vi "SGP Calculator.vi"(8 "End Flow":dbl, 9 "Flow Array":dbl[](array[numeric]), 10 "Start Index":i32, 11 "Resistance":dbl) -> (0 "End Flow Out":dbl, 2 "SGP":dbl, 3 "Start Flow":dbl)   [LabVIEW 2018, in "AnalysisSupport.lvlib"]
uses:
  AnalysisSupport.lvlib
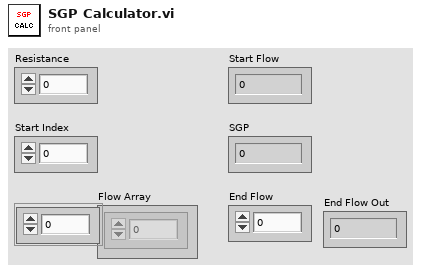
[diagram p1: front panel]
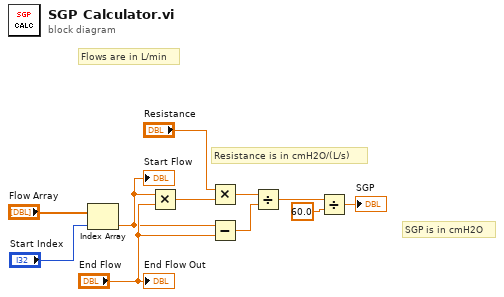
[diagram p0: block diagram]
diagram:
  # "Flows are in L/min"
  # "SGP is in cmH2O"
  # "Resistance is in cmH2O/(L/s)"
  n1 = Index Array(array="Flow Array", index="Start Index") -> (element=w8:dbl)
  "Start Flow" <- w8
  n2 = Multiply(x=w8, y="End Flow") -> (x*y=w6:dbl)
  n3 = Multiply(x="Resistance", y=w6) -> (x*y=w10:dbl)
  n4 = Subtract(x=w8, y="End Flow") -> (x-y=w11:dbl)
  n5 = Divide(x=w10, y=w11) -> (x/y=w2:dbl)
  n6 = Divide(x=w2, y=60.0) -> (x/y=→"SGP":dbl)
  "End Flow Out" <- "End Flow"
